vi "process_stim_chunky_NI.vi"(8 "error in (no error)":errorcluster) -> (0 "error out":errorcluster)   [LabVIEW 2010]
uses:
  typedefs/control_stim_enum.ctl
  typedefs/run_mode.ctl
  typedefs/device_parameters.ctl
  typedefs/protocol_parameters.ctl
  typedefs/free_run_parameters.ctl
  <vilib>/DAQmx/write.llb/DAQmx Write (Analog 1D DBL 1Chan NSamp).vi
  <vilib>/daqmx/miscellaneous.llb/DAQmx Fill In Error Info.vi
  Program Files/National Instruments/LabVIEW 2010/resource/objmgr/daqmx.rc
panel:
  out "Number of samples written":u32
  out "Write to queue":bool
  out "Internal stop":bool=TRUE
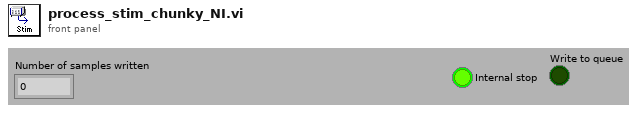
[diagram p1: front panel]
types:
  T1 = typedef "control_stim_enum.ctl" = enum16{"Init", "Stim Protocol", "Stim Free Run", "Stop", "Quit"}
  T2 = cluster{"Control stim Enum":T1, "variant":variant}
  T3 = typedef "run_mode.ctl" = enum32{"Protocol", "Free Run"}
  T4 = typedef "device_parameters.ctl" = cluster{"Triggered?":bool, "Shutter channel":tag, "Acquisition channels":tag, "Acquisition sample rate":dbl, "Read chunk size":i32, "Stimulation channel":tag, "Stimulation sample rate":dbl}
  T5 = typedef "protocol_parameters.ctl" = cluster{"Repetitions":dbl, "ON time":dbl, "OFF time":dbl, "Stim onset":dbl, "Stim frequency":dbl, "Pulse width":dbl, "Acquire before ON":dbl, "Acquire after ON":dbl, "Sync shutter to acquisition":bool}
  T6 = cluster{"Device parameters":T4, "Protocol parameters":T5}
  T7 = typedef "free_run_parameters.ctl" = cluster{"Stim onset":dbl, "Stim frequency":dbl, "Stim length":dbl, "Sync shutter to acquisition":bool}
  T8 = cluster{"Device parameters":T4, "Free run parameters":T7}
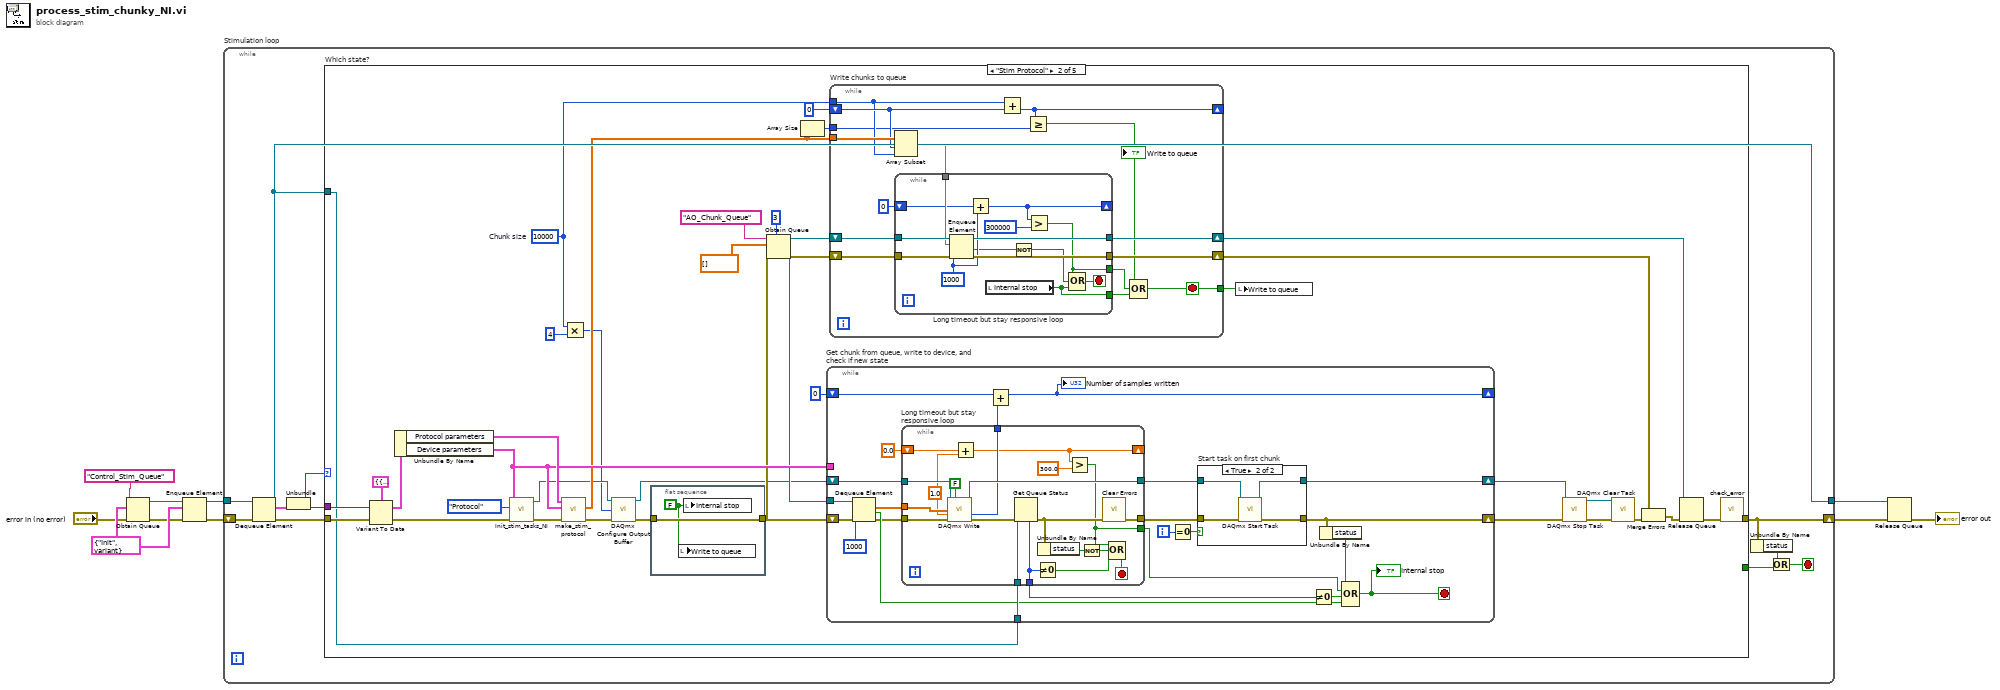
[diagram p0: block diagram]
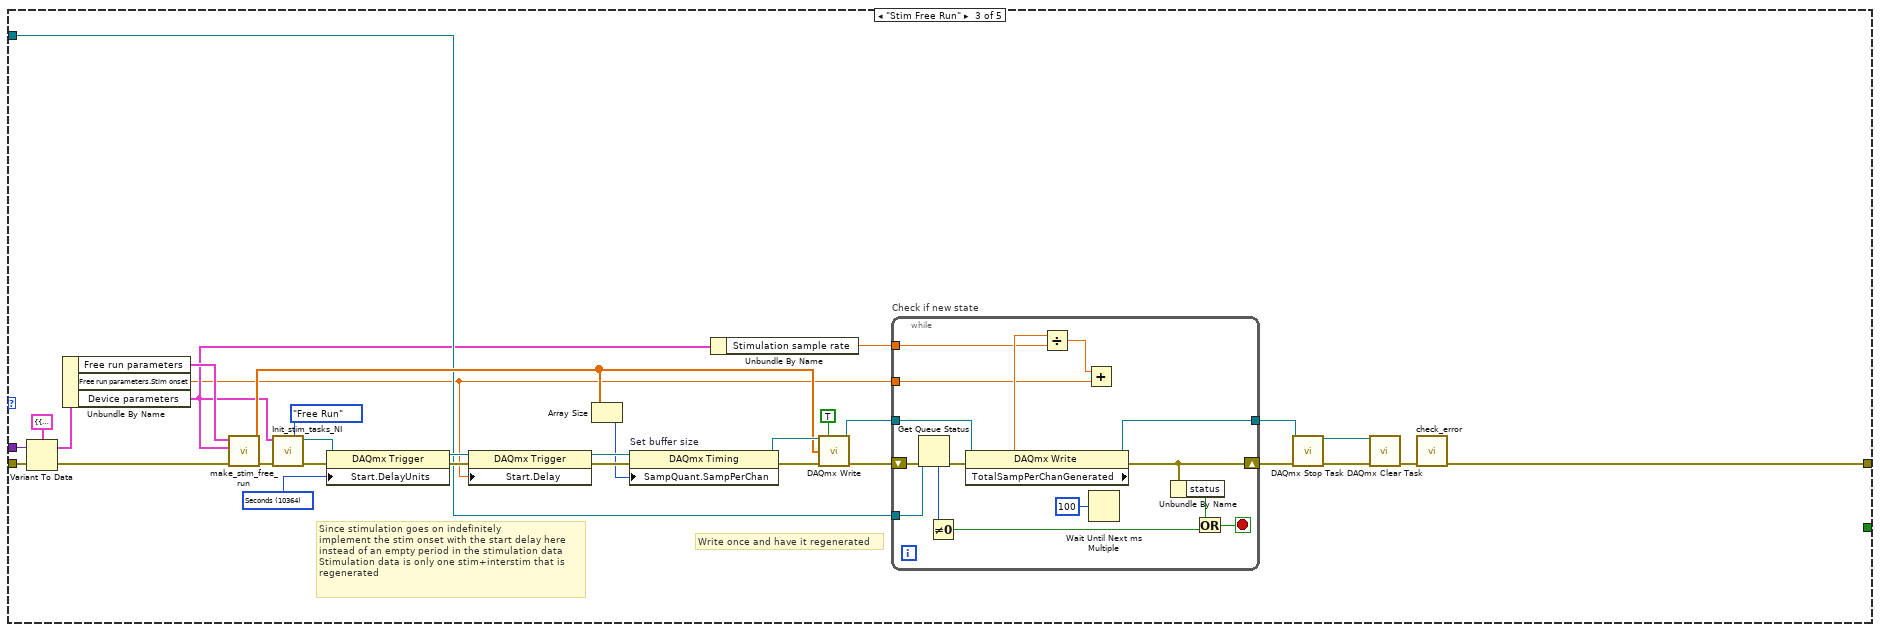
[diagram p4: hidden frame]
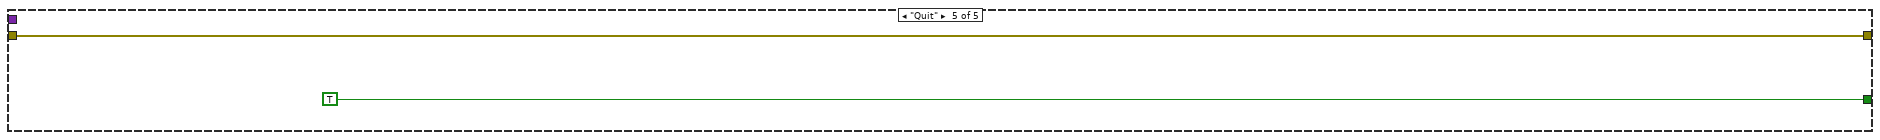
[diagram p6: hidden frame]
diagram:
  w10 = T2 {"Control stim Enum"=enum."Init", "variant"=variant} ("ControlDAQ state cluster")
  n1 = Obtain Queue(name (unnamed)="Control_Stim_Queue", element data type=w10, error in (no error)="error in (no error)") -> (queue out=w6:refnum<queue>, error out=w8:errorcluster)  [unwired: 2 in, 1 out]
  n2 = Enqueue Element(queue=w6, element=w10, error in (no error)=w8) -> (queue out=w7:refnum<queue>, error out=w9:errorcluster)  [unwired: 1 in, 1 out]
  n3 = while "Stimulation loop" {
    shift-right: [w15] -> w5
    shift-left: w9 -> [w20]
    tunnel: w7 -> [w21]
    tunnel: [w11] -> w4
    stop <- w13 stop-if-true
    n4 = Dequeue Element(queue=w21, error in (no error)=w20) -> (queue out=w11:refnum<queue>, element=w19:T2, error out=w17:errorcluster)  [unwired: 1 in, 1 out]
    n5 = Unbundle(w19) -> ("Control stim Enum"=w12:T1, "variant"=w18:variant)
    n6 = case "Which state?" shown="\"Stim Protocol\"" w12 {
      tunnel: w11 -> [_ w36 w151 _ _]
      tunnel: w18 -> [_ w60 w171 _ _]
      tunnel: w17 -> [w22 w59 w172 w188 w189]
      tunnel: [w22 w52 w148 w188 w189] -> w15
      tunnel: [_ _ _ _ TRUE] -> w16
      frame "Init", Default {
      }
      frame "Stim Protocol" {
        w26 = 10000  # Chunk size
        n7 = Variant To Data(error in=w59, Variant=w60, type=T6 {"Device parameters"={"Triggered?"=FALSE, "Shutter channel"="", "Acquisition channels"="", "Acquisition sample rate"=0.0, "Read chunk size"=0, "Stimulation channel"="", "Stimulation sample rate"=0.0}, "Protocol parameters"={"Repetitions"=0.0, "ON time"=0.0, "OFF time"=0.0, "Stim onset"=0.0, "Stim frequency"=0.0, "Pulse width"=0.0, "Acquire before ON"=0.0, "Acquire after ON"=0.0, "Sync shutter to acquisition"=FALSE}}) -> (error out=w58:errorcluster, data=w55:T6)
        n8 = Unbundle By Name(w55) -> ("Protocol parameters"=w54:T5, "Device parameters"=w51:T4)
        n9 = call "Init_stim_tasks_NI.vi"("error in"=w58, "Run mode"=run_mode."Protocol", "Device parameters"=w51) -> ("error out"=w57:errorcluster, "Stim task out"=w28:refnum<k21>)  [unwired: 5 in]
        n10 = call "make_stim_protocol.vi"("Error in"=w57, "Device parameters"=w51, "Protocol parameters"=w54) -> ("Error out"=w30:errorcluster, "Stim array"=w45:dbl[])  [unwired: 7 in]
        n11 = Multiply(x=w26, y=4) -> (x*y=w24:i32)
        n12 = call <vilib>:"DAQmx Configure Output Buffer.vi"("task/channels in"=w28, "buffer size (in samples per channel)"=w24, "error in"=w30) -> ("task out"=w27:refnum<k21>, "error out"=w29:errorcluster)  [unwired: 11 in]
        n13 = flat-sequence {
          tunnel: w29 -> [w62]
          tunnel: [w62] -> w37
          frame #0 {
            w61 = FALSE ("internal stop")
            n14 = local write "Write to queue"(w61) -> ()
            n15 = local write "Internal stop"(w61) -> ()
          }
        }
        n16 = Obtain Queue(max queue size (-1, unlimited)=3, name (unnamed)="AO_Chunk_Queue", element data type=dbl[] [], error in (no error)=w37) -> (queue out=w43:refnum<queue>, error out=w48:errorcluster)  [unwired: 1 in, 1 out]
        n17 = Array Size(array=w45) -> (size(s)=w44:i32)
        n18 = while "Get chunk from queue, write to device, and check if new state" {
          shift-right: [w95] -> w35
          shift-left: w37 -> [w114]
          tunnel: w51 -> [_]
          tunnel: w43 -> [w113]
          tunnel: w36 -> [w110]
          shift-right: [w105] -> w33
          shift-left: w27 -> [w102]
          shift-right: [w104] -> _
          shift-left: u32 0 -> [w98]
          i -> [w112]
          stop <- w107 stop-if-true
          n19 = Dequeue Element(queue=w113, timeout in ms (-1)=1000, error in (no error)=w114) -> (element=w100:dbl[], timed out?=w106:bool, error out=w103:errorcluster)  [unwired: 1 out]
          n20 = while "Long timeout but stay responsive loop" {
            tunnel: w110 -> [w134]
            tunnel: [w122] -> w109
            tunnel: w103 -> [w133]
            tunnel: w102 -> [w132]
            tunnel: [w131] -> w101
            tunnel: w100 -> [w130]
            tunnel: [w128] -> w99
            tunnel: [w121] -> w96
            shift-right: [w124] -> _
            shift-left: 0.0 -> [w125]
            tunnel: [w115] -> w92
            stop <- w116 stop-if-true
            w126 = 1.0 ("timeout")
            n21 = call-poly <vilib>:"DAQmx Write.vi"("task/channels in"=w132, "auto start"=FALSE, "data"=w130, "timeout"=w126, "error in"=w133) -> ("task out"=w131:refnum<k21>, "number of samples written per channel"=w128:u32, "error out"=w127:errorcluster)  [unwired: 8 in]
            n22 = Add(x=w125, y=w126) -> (x+y=w124:dbl)
            n23 = Get Queue Status(queue=w134, error in (no error)=w127) -> (error out=w120:errorcluster, # elements in queue=w122:i32)  [unwired: 1 in, 6 out]
            n24 = Not Equal To 0?(x=w122) -> (x != 0?=w117:bool)
            n25 = Unbundle By Name(w120) -> ("status"=w119:bool)
            n26 = Greater?(x=w124, y=300.0) -> (0:w115:bool)
            n27 = Not(x=w119) -> (.not. x?=w118:bool)
            n28 = call <vilib>:"Clear Errors.vi"("error in (no error)"=w120) -> ("error out"=w121:errorcluster)  [unwired: 6 in]
            n29 = Compound Arithmetic op=OR(w115, w118, w117) -> (w116:bool)
          }
          n30 = Add(x=w98, y=w99) -> (x+y=w104:u32)
          "Number of samples written" <- w104
          n31 = Equal To 0?(x=w112) -> (x = 0?=w111:bool)
          n32 = case "Start task on first chunk" shown="True" w111 {
            tunnel: w96 -> [w135 w140]
            tunnel: w101 -> [w136 w138]
            tunnel: [w135 w139] -> w95
            tunnel: [w136 w137] -> w105
            frame False {
            }
            frame True {
              n33 = call <vilib>:"DAQmx Start Task.vi"("task/channels in"=w138, "error in"=w140) -> ("task out"=w137:refnum<k21>, "error out"=w139:errorcluster)  [unwired: 12 in]
            }
          }
          n34 = Not Equal To 0?(x=w109) -> (x != 0?=w108:bool)
          n35 = Unbundle By Name(w95) -> ("status"=w93:bool)
          n36 = Compound Arithmetic op=OR(w93, w92, w108, w106) -> (w107:bool)
          "Internal stop" <- w107
        }
        n37 = while "Write chunks to queue" {
          shift-right: [w68] -> w42
          shift-left: w48 -> [w74]
          tunnel: w45 -> [w77]
          shift-right: [w72] -> _
          shift-left: 0 -> [w76]
          tunnel: w26 -> [w75]
          shift-right: [w70] -> w38
          shift-left: w43 -> [w73]
          tunnel: w44 -> [w71]
          tunnel: [w66] -> w23
          stop <- w66 stop-if-true
          n38 = Array Subset(array=w77, index=w76, length=w75) -> (w69:dbl[])
          n39 = while "Long timeout but stay responsive loop" {
            tunnel: w74 -> [w91]
            tunnel: w73 -> [w90]
            tunnel: [w89] -> w70
            tunnel: w69 -> [w88]
            tunnel: [w87] -> w68
            shift-right: [w84] -> _
            shift-left: 0 -> [w85]
            tunnel: [w79] -> w65
            tunnel: [w78] -> w63
            stop <- w82 stop-if-true
            w86 = 1000 ("timeout in ms (-1)")
            n40 = Enqueue Element(queue=w90, element=w88, timeout in ms (-1)=w86, error in (no error)=w91) -> (queue out=w89:refnum<queue>, timed out?=w81:bool, error out=w87:errorcluster)
            n41 = Add(x=w85, y=w86) -> (x+y=w84:i32)
            n42 = local read "Internal stop"() -> (w79:bool)
            n43 = Not(x=w81) -> (.not. x?=w80:bool)
            n44 = Greater?(x=w84, y=300000) -> (0:w78:bool)
            n45 = Compound Arithmetic op=OR(w78, w80, w79) -> (w82:bool)
          }
          n46 = Add(x=w75, y=w76) -> (x+y=w72:i32)
          n47 = Greater Or Equal?(x=w72, y=w71) -> (x >= y?=w64:bool)
          "Write to queue" <- w64
          n48 = Compound Arithmetic op=OR(w64, w63, w65) -> (w66:bool)
        }
        n49 = local write "Write to queue"(w23) -> ()
        n50 = call <vilib>:"DAQmx Stop Task.vi"("task/channels in"=w33, "error in"=w35) -> ("task out"=w32:refnum<k21>, "error out"=w34:errorcluster)  [unwired: 12 in]
        n51 = call <vilib>:"DAQmx Clear Task.vi"("task in"=w32, "error in"=w34) -> ("error out"=w41:errorcluster)  [unwired: 13 in]
        n52 = Merge Errors(w42, w41) -> (w40:errorcluster)
        n53 = Release Queue(queue=w38, error in (no error)=w40) -> (error out=w39:errorcluster)  [unwired: 1 in, 2 out]
        n54 = call "check_error.vi"("error in"=w39) -> ("error out"=w52:errorcluster)  [unwired: 10 in]
      }
      frame "Stim Free Run" {
        w166 = 10364 items=["Sample Clock Periods"=10286, "Seconds"=10364, "Ticks"=10304] ("Start.DelayUnits")
        # "Write once and have it regenerated"
        # "Since stimulation goes on indefinitely\nimplement the stim onset with the start delay here\ninstead of an empty period in the stimulation data\nStimulation data is only one stim+interstim that is\nregenerated"
        n55 = Variant To Data(error in=w172, Variant=w171, type=T8 {"Device parameters"={"Triggered?"=FALSE, "Shutter channel"="", "Acquisition channels"="", "Acquisition sample rate"=0.0, "Read chunk size"=0, "Stimulation channel"="", "Stimulation sample rate"=0.0}, "Free run parameters"={"Stim onset"=0.0, "Stim frequency"=0.0, "Stim length"=0.0, "Sync shutter to acquisition"=FALSE}} ("output cluster")) -> (error out=w161:errorcluster, data=w169:T8)
        n56 = Unbundle By Name(w169) -> ("Free run parameters"=w162:T7, "Free run parameters.Stim onset"=w145:dbl, "Device parameters"=w147:T4)
        n57 = call "make_stim_free_run.vi"("error in"=w161, "Device parameters"=w147, "Free run parameters"=w162) -> ("error out"=w160:errorcluster, "Stim array"=w154:dbl[])  [unwired: 7 in]
        n58 = call "Init_stim_tasks_NI.vi"("error in"=w160, "Run mode"=run_mode."Free Run", "Device parameters"=w147) -> ("error out"=w164:errorcluster, "Stim task out"=w163:refnum<k21>)  [unwired: 5 in]
        n59 = property class="DAQmx Trigger"(reference=w163, error in=w164, "Start.DelayUnits"=w166) -> (reference out=w167:refnum<k21>, error out=w168:errorcluster)
        n60 = property class="DAQmx Trigger"(reference=w167, error in=w168, "Start.Delay"=w145) -> (reference out=w158:refnum<k21>, error out=w159:errorcluster)
        n61 = Array Size(array=w154) -> (size(s)=w157:i32)
        n62 = property on="Set buffer size" class="DAQmx Timing"(reference=w158, error in=w159, "SampQuant.SampPerChan"=w157) -> (reference out=w155:refnum<k21>, error out=w156:errorcluster)
        n63 = Unbundle By Name(w147) -> ("Stimulation sample rate"=w146:dbl)
        n64 = call-poly <vilib>:"DAQmx Write.vi"("task/channels in"=w155, "auto start"=TRUE, "data"=w154, "error in"=w156) -> ("task out"=w150:refnum<k21>, "error out"=w152:errorcluster)  [unwired: 9 in, 1 out]
        n65 = while "Check if new state" {
          tunnel: w151 -> [w186]
          shift-right: [w179] -> w144
          shift-left: w152 -> [w187]
          tunnel: w150 -> [w176]
          tunnel: [w175] -> w141
          tunnel: w146 -> [w177]
          tunnel: w145 -> [w174]
          stop <- w182 stop-if-true
          n66 = Get Queue Status(queue=w186, error in (no error)=w187) -> (error out=w180:errorcluster, # elements in queue=w185:i32)  [unwired: 1 in, 6 out]
          n67 = Not Equal To 0?(x=w185) -> (x != 0?=w184:bool)
          n68 = property class="DAQmx Write"(reference=w176, error in=w180) -> (reference out=w175:refnum<k21>, error out=w179:errorcluster, "TotalSampPerChanGenerated"=w178:dbl)
          n69 = Divide(x=w178, y=w177) -> (x/y=w173:dbl)
          n70 = Add(x=w173, y=w174) -> ()  [unwired: 1 out]
          n71 = Wait Until Next ms Multiple(millisecond multiple=u32 100) -> ()  [unwired: 1 out]
          n72 = Unbundle By Name(w179) -> ("status"=w183:bool)
          n73 = Or(x=w183, y=w184) -> (x .or. y?=w182:bool)
        }
        n74 = call <vilib>:"DAQmx Stop Task.vi"("task/channels in"=w141, "error in"=w144) -> ("task out"=w142:refnum<k21>, "error out"=w143:errorcluster)  [unwired: 12 in]
        n75 = call <vilib>:"DAQmx Clear Task.vi"("task in"=w142, "error in"=w143) -> ("error out"=w149:errorcluster)  [unwired: 13 in]
        n76 = call "check_error.vi"("error in"=w149) -> ("error out"=w148:errorcluster)  [unwired: 10 in]
      }
      frame "Stop" {
      }
      frame "Quit" {
      }
    }
    n77 = Unbundle By Name(w15) -> ("status"=w14:bool)
    n78 = Or(x=w14, y=w16) -> (x .or. y?=w13:bool)
  }
  n79 = Release Queue(queue=w4, error in (no error)=w5) -> (error out=→"error out":errorcluster)  [unwired: 1 in, 2 out]
